vi "ConfigSignal.vi"(0 "reference in":refnum<class "LCR_BK891.lvclass">, 5 "Signal Frequency (1000 Hz)":dbl=1000.0 format="%#_4g", 7 "Signal Level (0:0.5 Vrms)":u8(ring) items=["0.5Vrms", "1Vrms"], 11 "error in (no error)":errorcluster) -> (4 "reference in":refnum<class "LCR_BK891.lvclass">, 15 "error out":errorcluster)   [LabVIEW 2022 SP3, in "LCR_BK891.lvlib" / "LCR_BK891.lvclass"]
uses:
  LCR_BK891.lvclass
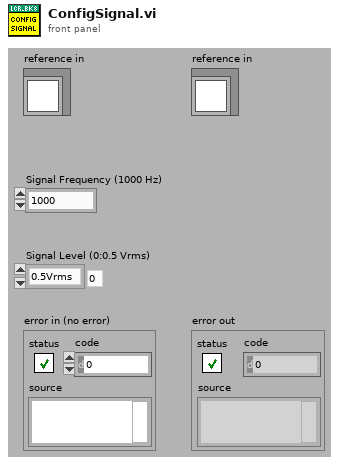
[diagram p1: front panel]
types:
  T1 = typedef "LCR_BK891.lvlib/LCR_BK891.lvclass/ObjectAttributes.ctl" = cluster{"Config":T2, "VISA Ref":refnum<visa-resource-name>, "Function":u16, "Range":u16, "Measurement Speed":u16, "Signal Frequency":dbl, "Signal Level":u8, "Measured Primary Reading":dbl, "Measured Secondary Reading":dbl}
  T2 = typedef "LCR_BK891.lvlib/LCR_BK891.lvclass/Config.ctl" = cluster{"VISA":refnum<visa-resource-name>}
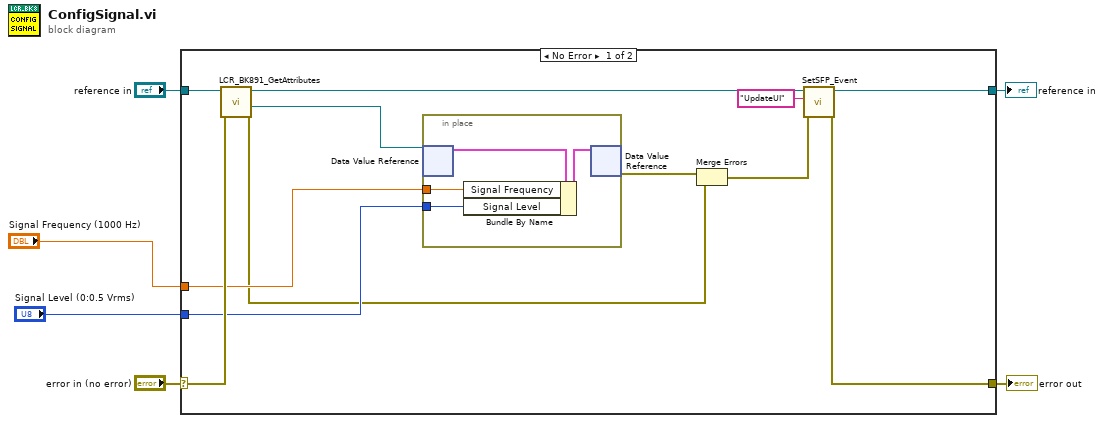
[diagram p0: block diagram]
diagram:
  n1 = case shown="No Error" "error in (no error)" {
    selector: "error in (no error)" -> [w18 w24]
    tunnel: [w13 w24] -> w5
    tunnel: [w14 w23] -> w3
    tunnel: "reference in" -> [w17 w23]
    tunnel: "Signal Frequency (1000 Hz)" -> [w9 _]
    tunnel: "Signal Level (0:0.5 Vrms)" -> [w8 _]
    frame No Error {
      n2 = call "LCR_BK891_GetAttributes.vi"("error in (no error)"=w18, "reference in"=w17) -> ("error out"=w7:errorcluster, "DataRef"=w16:refnum<data-value>, "reference out"=w15:refnum<class "LCR_BK891.lvclass">)  [unwired: 6 in, 1 out]
      n3 = in-place {
        in-place-border: w9 -> [w20]
        in-place-border: w8 -> [w19]
        n4 = in-place-dvr #1(w16) -> (w22:T1)  [unwired: 1 out]
        n5 = Bundle By Name(cluster=w22, "Signal Frequency"=w20, "Signal Level"=w19) -> (w21:T1)
        n6 = in-place-dvr #1(w21) -> (w12:errorcluster)  [unwired: 1 out]
      }
      n7 = Merge Errors(w12, w7) -> (w11:errorcluster)
      n8 = call-dynamic "SetSFP_Event.vi"("error in (no error)"=w11, "msg"="UpdateUI", "reference in"=w15) -> ("error out"=w13:errorcluster, "reference out"=w14:refnum<class "LCR_BK891.lvclass">)  [unwired: 7 in]
    }
    frame Error {
    }
  }
  "error out" <- w5
  "reference in" <- w3
